vi "Start.vi"(8 "error in (no error)":errorcluster, 11 "Motor-DAQmx in":refnum<class "Motor-DAQmx.lvclass">) -> (0 "error out":errorcluster, 3 "Motor-DAQmx out":refnum<class "Motor-DAQmx.lvclass">)   [LabVIEW 2013, in "PowderDeposition.lvlib" / "Motor-DAQmx.lvclass"]
uses:
  Motor-DAQmx.lvclass
  Motor-DAQmx.lvclass/Motor-DAQmx.ctl
  <vilib>/DAQmx/write.llb/DAQmx Write (Digital Bool 1Line 1Point).vi
  <vilib>/DAQmx/miscellaneous.llb/DAQmx Fill In Error Info.vi
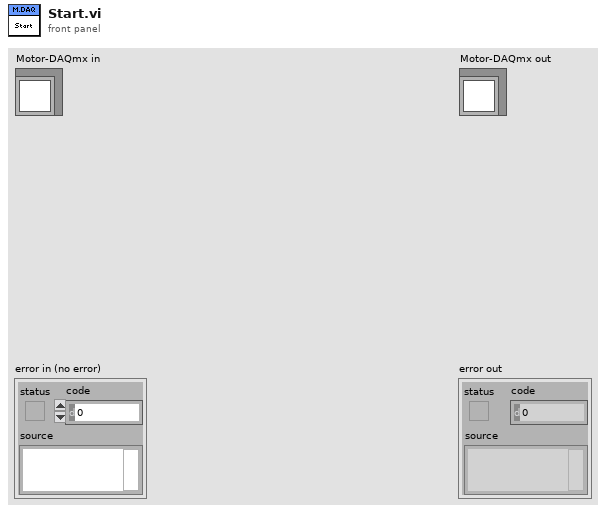
[diagram p1: front panel]
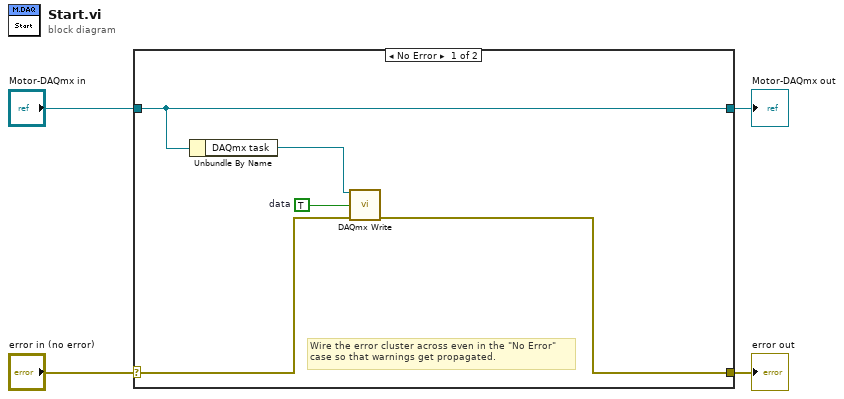
[diagram p0: block diagram]
diagram:
  n1 = case shown="No Error" "error in (no error)" {
    selector: "error in (no error)" -> [w6 w11]
    tunnel: [w5 w11] -> w3
    tunnel: [w9 w10] -> w1
    tunnel: "Motor-DAQmx in" -> [w9 w10]
    frame No Error {
      w7 = TRUE  # data
      # "Wire the error cluster across even in the \"No Error\"\ncase so that warnings get propagated."
      n2 = Unbundle By Name(w9) -> ("DAQmx task"=w8:refnum<k21>)
      n3 = call-poly <vilib>:"DAQmx Write.vi"("task/channels in"=w8, "data"=w7, "error in"=w6) -> ("error out"=w5:errorcluster)  [unwired: 10 in, 2 out]
    }
    frame Error {
    }
  }
  "error out" <- w3
  "Motor-DAQmx out" <- w1
